vi "String To Array Test.vi"() -> ()   [LabVIEW 2021, in "Test Files.lvlib"]
uses:
  Test Files.lvlib
  CustomSortPath.lvlib
  <vilib>/addons/_JKI Toolkits/Caraya/classes/Test/Test.lvclass
  <vilib>/addons/_JKI Toolkits/Caraya/classes/Assert/Assert.lvclass
  <vilib>/addons/_JKI Toolkits/Caraya/classes/Assert/Assert Equal Value_Variant.vi
panel:
  out "error out":errorcluster
  in  "error in (no error)":errorcluster
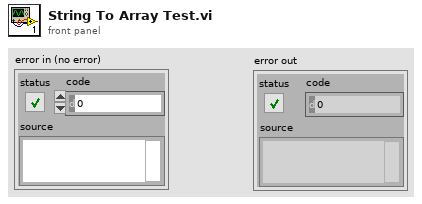
[diagram p1: front panel]
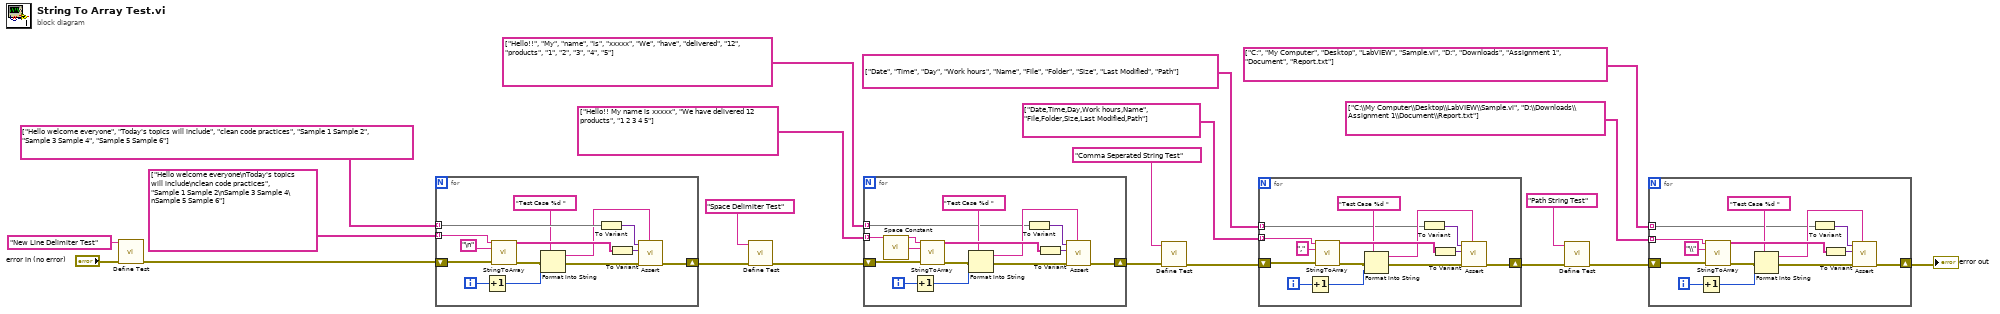
[diagram p0: block diagram]
diagram:
  n1 = call <vilib>:"Define Test.vi"("error in (no error)"="error in (no error)", "Label (VI Title)"="New Line Delimiter Test") -> ("error out"=w19:errorcluster)  [unwired: 8 in, 1 out]
  n2 = for {
    tunnel: string[] ["Hello welcome everyone\nToday's topics will include\nclean code practices", "Sample 1 Sample 2\nSample 3 Sample 4\nSample 5 Sample 6"] -> [w33] mode=indexing
    tunnel: string[][] [["Hello welcome everyone", "Today's topics will include", "clean code practices"], ["Sample 1 Sample 2", "Sample 3 Sample 4", "Sample 5 Sample 6"]] ("appended array") -> [w30] mode=indexing
    shift-right: [w22] -> w16
    shift-left: w19 -> [w35]
    i -> [w28]
    n3 = Increment(x=w28) -> (x+1=w26:i32)
    n4 = call "StringToArray.vi"("String"=w33, "delimiter (Tab)"="\n", "error in (no error)"=w35) -> ("1DArray"=w32:string[], "error out"=w27:errorcluster)  [unwired: 11 in]
    n5 = Format Into String(format string="Test Case %d ", error in=w27, w26) -> (resulting string=w24:string, error out=w23:errorcluster)  [unwired: 1 in]
    n6 = To Variant(anything=w30) -> (Variant=w29:variant)
    n7 = To Variant(anything=w32) -> (Variant=w31:variant)
    n8 = call-poly <vilib>:"Assert.vi"("Label"=w24, "error in (no error)"=w23, "Y"=w31, "X"=w29) -> ("error out"=w22:errorcluster)  [unwired: 6 in, 1 out]
  }
  n9 = call <vilib>:"Define Test.vi"("error in (no error)"=w16, "Label (VI Title)"="Space Delimiter Test") -> ("error out"=w14:errorcluster)  [unwired: 8 in, 1 out]
  n10 = for {
    shift-right: [w39] -> w11
    shift-left: w14 -> [w49]
    tunnel: string[][] [["Hello!!", "My", "name", "is", "xxxxx"], ["We", "have", "delivered", "12", "products"], ["1", "2", "3", "4", "5"]] ("appended array") -> [w38] mode=indexing
    tunnel: string[] ["Hello!! My name is xxxxx", "We have delivered 12 products", "1 2 3 4 5"] -> [w37] mode=indexing
    i -> [w45]
    n11 = call <vilib>:"Space Constant.vi"() -> ("String"=w36:string)
    n12 = Increment(x=w45) -> (x+1=w43:i32)
    n13 = call "StringToArray.vi"("String"=w37, "delimiter (Tab)"=w36, "error in (no error)"=w49) -> ("1DArray"=w48:string[], "error out"=w44:errorcluster)  [unwired: 11 in]
    n14 = Format Into String(format string="Test Case %d ", error in=w44, w43) -> (resulting string=w41:string, error out=w40:errorcluster)  [unwired: 1 in]
    n15 = To Variant(anything=w38) -> (Variant=w46:variant)
    n16 = To Variant(anything=w48) -> (Variant=w47:variant)
    n17 = call-poly <vilib>:"Assert.vi"("Label"=w41, "error in (no error)"=w40, "Y"=w47, "X"=w46) -> ("error out"=w39:errorcluster)  [unwired: 6 in, 1 out]
  }
  n18 = call <vilib>:"Define Test.vi"("error in (no error)"=w11, "Label (VI Title)"="Comma Seperated String Test") -> ("error out"=w9:errorcluster)  [unwired: 8 in, 1 out]
  n19 = for {
    shift-right: [w53] -> w5
    shift-left: w9 -> [w63]
    tunnel: string[] ["Date,Time,Day,Work hours,Name", "File,Folder,Size,Last Modified,Path"] -> [w52] mode=indexing
    tunnel: string[][] [["Date", "Time", "Day", "Work hours", "Name"], ["File", "Folder", "Size", "Last Modified", "Path"]] ("appended array") -> [w50] mode=indexing
    i -> [w59]
    n20 = Increment(x=w59) -> (x+1=w57:i32)
    n21 = call "StringToArray.vi"("String"=w52, "delimiter (Tab)"=",", "error in (no error)"=w63) -> ("1DArray"=w62:string[], "error out"=w58:errorcluster)  [unwired: 11 in]
    n22 = Format Into String(format string="Test Case %d ", error in=w58, w57) -> (resulting string=w55:string, error out=w54:errorcluster)  [unwired: 1 in]
    n23 = To Variant(anything=w50) -> (Variant=w60:variant)
    n24 = To Variant(anything=w62) -> (Variant=w61:variant)
    n25 = call-poly <vilib>:"Assert.vi"("Label"=w55, "error in (no error)"=w54, "Y"=w61, "X"=w60) -> ("error out"=w53:errorcluster)  [unwired: 6 in, 1 out]
  }
  n26 = call <vilib>:"Define Test.vi"("error in (no error)"=w5, "Label (VI Title)"="Path String Test") -> ("error out"=w4:errorcluster)  [unwired: 8 in, 1 out]
  n27 = for {
    shift-right: [w67] -> w2
    shift-left: w4 -> [w77]
    tunnel: string[] ["C:\\My Computer\\Desktop\\LabVIEW\\Sample.vi", "D:\\Downloads\\Assignment 1\\Document\\Report.txt"] -> [w64] mode=indexing
    tunnel: string[][] [["C:", "My Computer", "Desktop", "LabVIEW", "Sample.vi"], ["D:", "Downloads", "Assignment 1", "Document", "Report.txt"]] ("appended array") -> [w65] mode=indexing
    i -> [w73]
    n28 = Increment(x=w73) -> (x+1=w71:i32)
    n29 = call "StringToArray.vi"("String"=w64, "delimiter (Tab)"="\\", "error in (no error)"=w77) -> ("1DArray"=w76:string[], "error out"=w72:errorcluster)  [unwired: 11 in]
    n30 = Format Into String(format string="Test Case %d ", error in=w72, w71) -> (resulting string=w69:string, error out=w68:errorcluster)  [unwired: 1 in]
    n31 = To Variant(anything=w65) -> (Variant=w74:variant)
    n32 = To Variant(anything=w76) -> (Variant=w75:variant)
    n33 = call-poly <vilib>:"Assert.vi"("Label"=w69, "error in (no error)"=w68, "Y"=w75, "X"=w74) -> ("error out"=w67:errorcluster)  [unwired: 6 in, 1 out]
  }
  "error out" <- w2
